vi "Railway-Crossing_vFinal_1.vi"() -> ()   [LabVIEW 2021]
uses:
  <vilib>/Utility/error.llb/DialogType.ctl
  <vilib>/DAQmx/write.llb/DAQmx Write (Counter Frequency 1Chan 1Samp).vi
  <vilib>/DAQmx/create/channels.llb/DAQmx Create Channel (CO-Pulse Generation-Frequency).vi
  <vilib>/DAQmx/configure/timing.llb/DAQmx Timing (Implicit).vi
  <vilib>/DAQmx/miscellaneous.llb/DAQmx Fill In Error Info.vi
panel:
  in  "stop 2":bool caption="stop"
  out "Car Counter 2":dbl
  out "Peak/Off-Peak":bool
  out "Car Counter":dbl
  out "Elapsed Time":dbl format="%#.0p"
  out "Time of Day":string
  out "Servo 2":bool
  out "Servo":bool
  in  "stop":bool
  out "Train":bool
  out "Train 2":bool
  out "Trainf":bool
  out "GREEN 2":bool
  out "YELLOW 2":bool
  out "RED  2":bool
  out "GREEN 1":bool
  out "YELLOW 1":bool
  out "GREEN":bool
  out "YELLOW":bool
  out "RED1":bool
  out "RED":bool
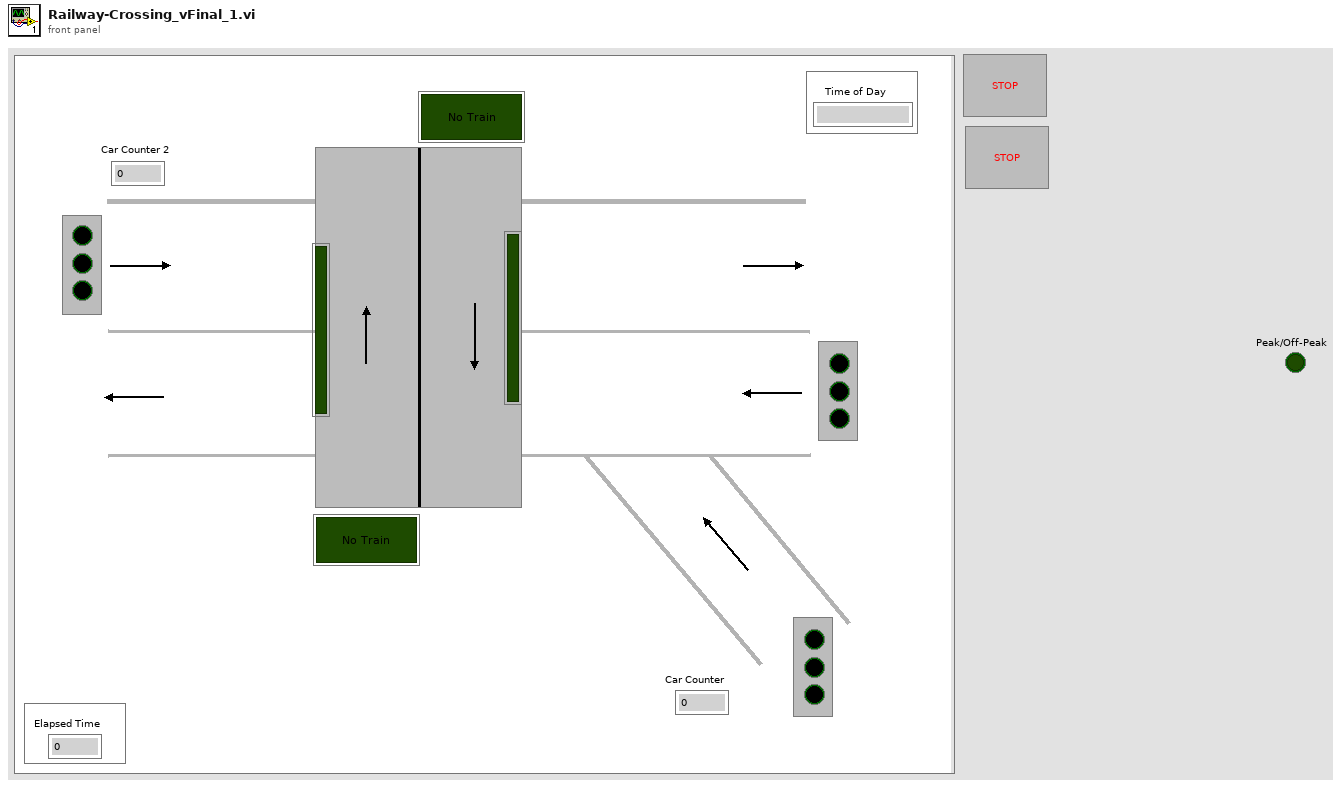
[diagram p1: front panel]
types:
  T1 = typedef "DialogType.ctl" = u16
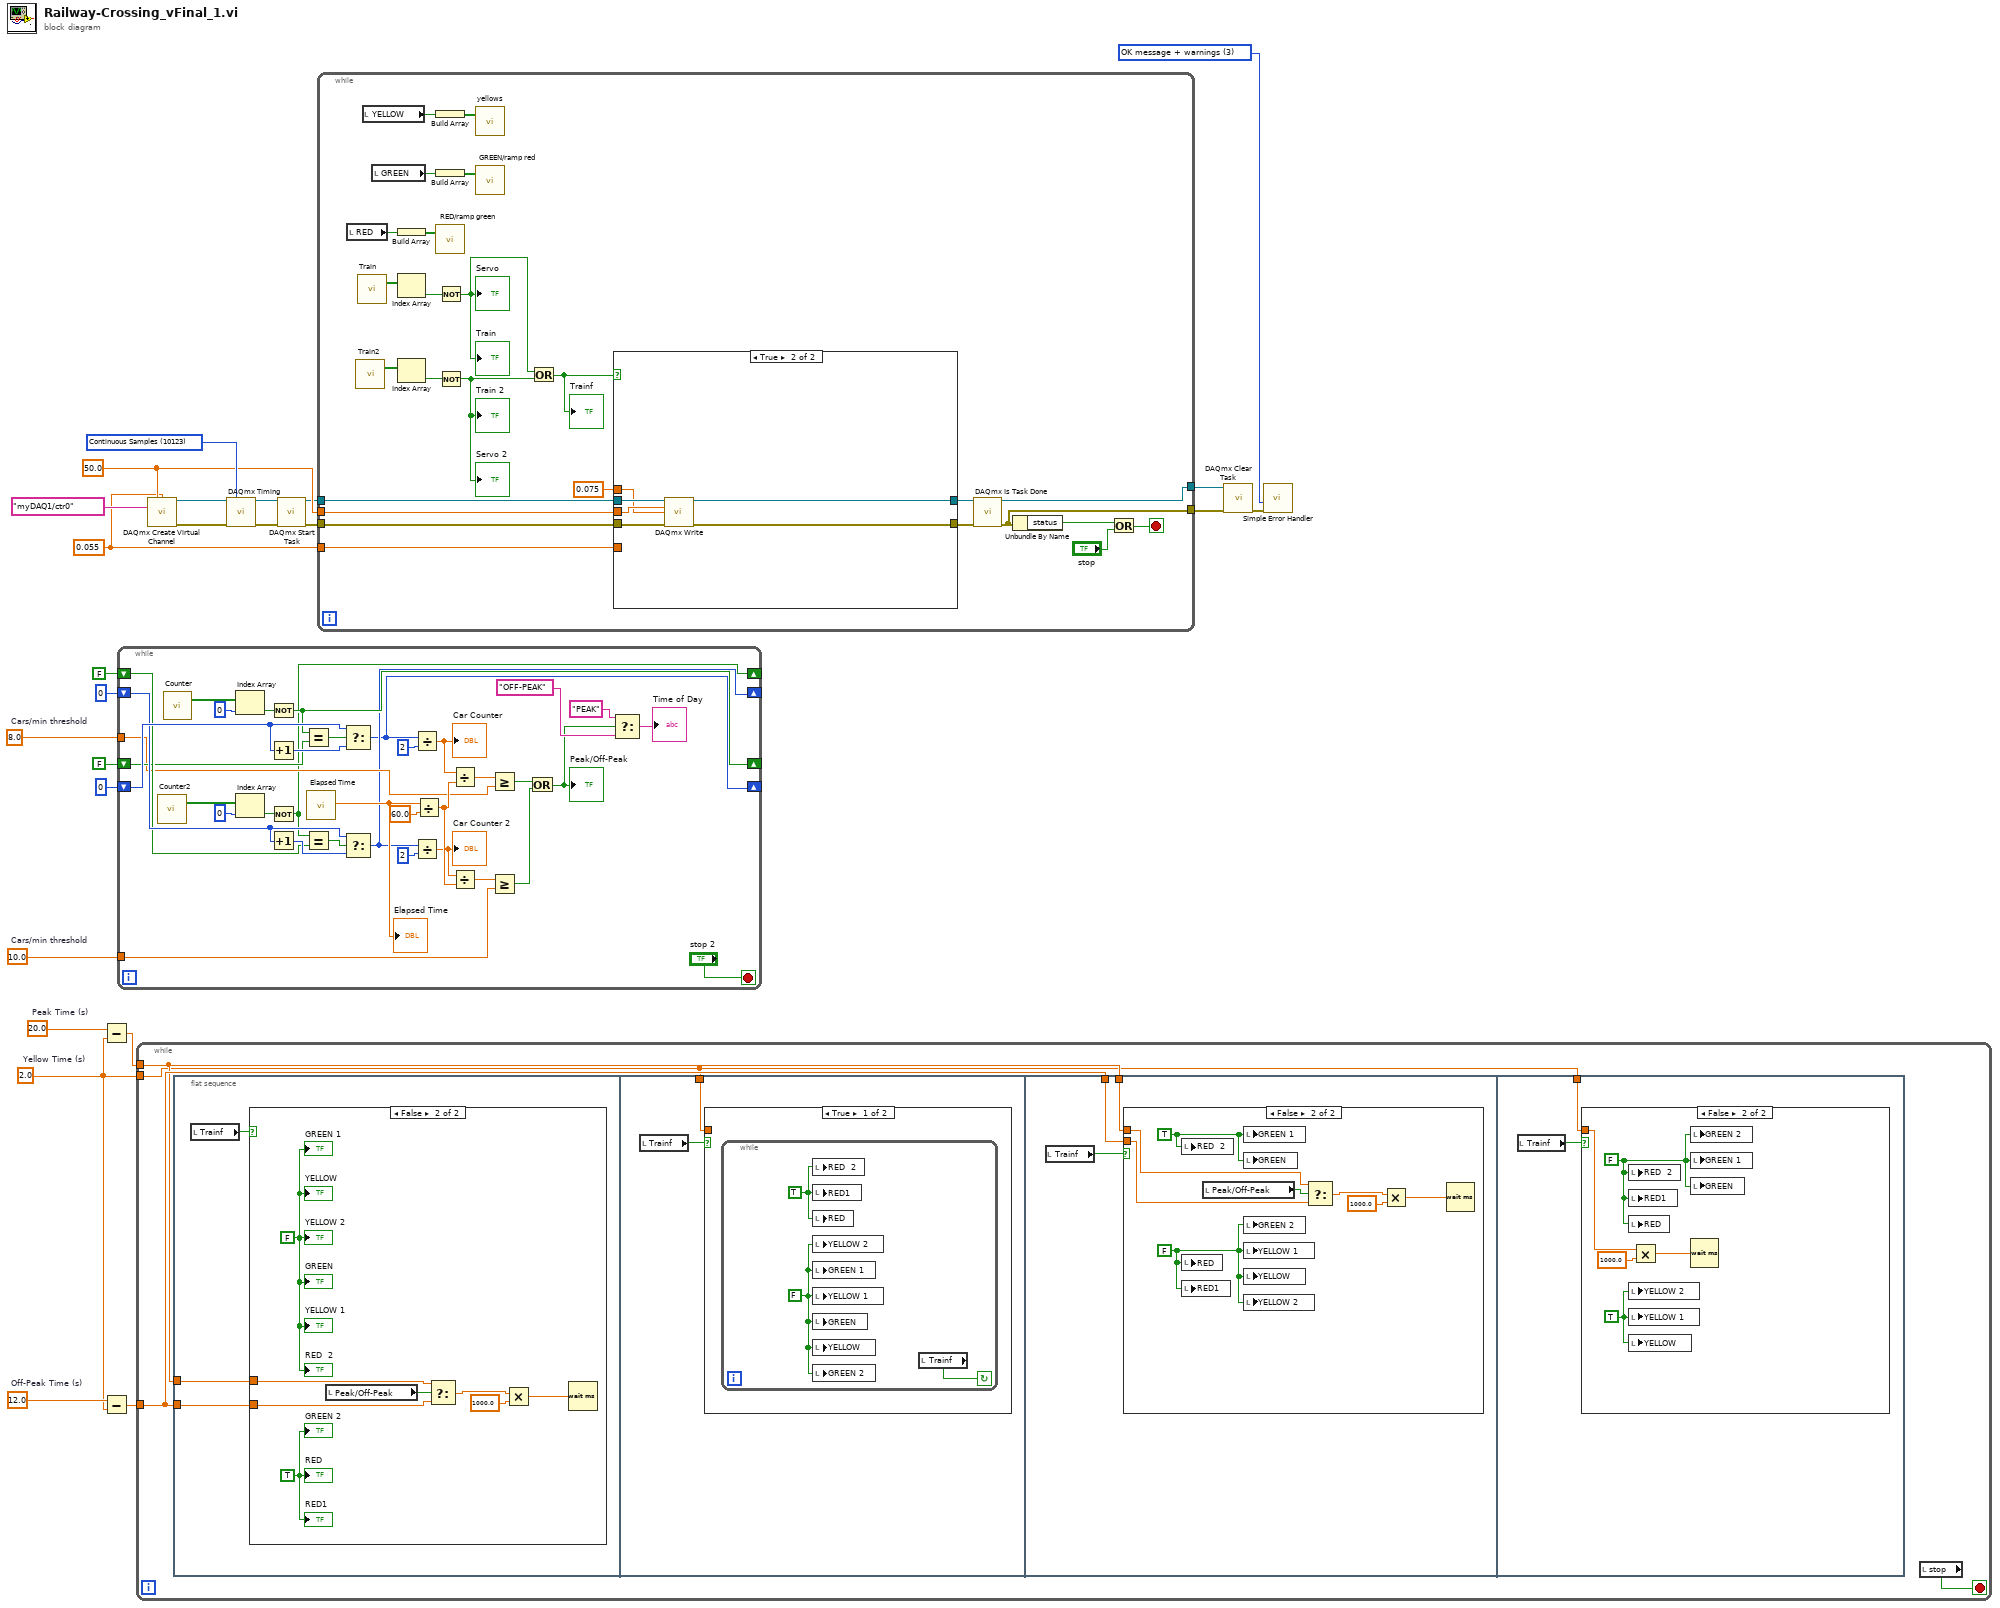
[diagram p0: block diagram]
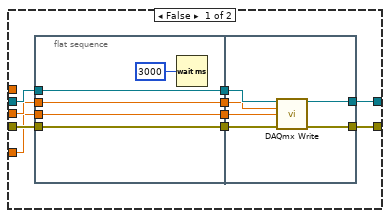
[diagram p2: hidden frame]
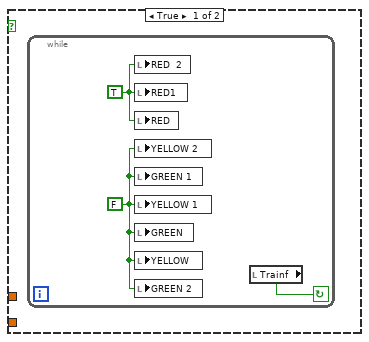
[diagram p3: hidden frame]
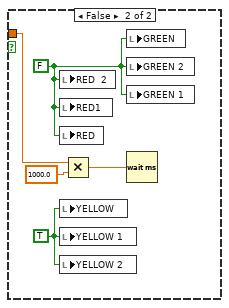
[diagram p4: hidden frame]
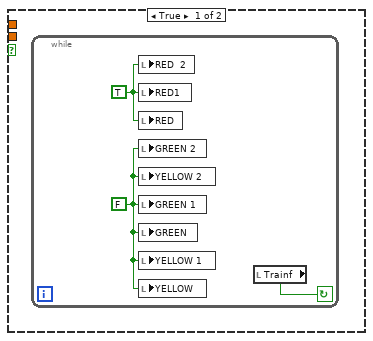
[diagram p5: hidden frame]
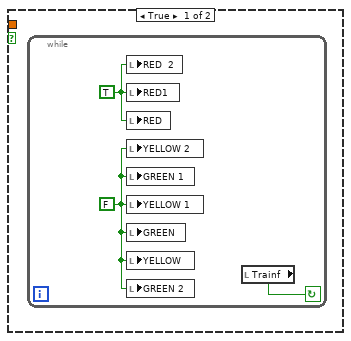
[diagram p6: hidden frame]
diagram:
  w2 = 10.0  # Cars/min threshold
  w1 = 8.0  # Cars/min threshold
  w10 = T1 3 items=["no dialog", "OK message", "continue or stop message", "OK message + warnings", "continue/stop + warnings"] ("type of dialog (OK msg:1)")
  w7 = 0.055 ("Duty Cycle")
  w14 = 50.0 ("Frequency")
  w16 = 10123 items=["Finite Samples"=10178, "Continuous Samples"=10123] ("sample mode")
  w23 = 20.0  # Peak Time (s)
  w22 = 2.0  # Yellow Time (s)
  w24 = 12.0  # Off-Peak Time (s)
  n1 = Subtract(x=w23, y=w22) -> (x-y=w21:dbl)
  n2 = Subtract(x=w24, y=w22) -> (x-y=w25:dbl)
  n3 = while {
    shift-right: [w32] -> _
    shift-left: FALSE -> [w37]
    shift-right: [w31] -> _
    shift-left: 0 -> [w38]
    shift-right: [w33] -> _
    shift-left: FALSE -> [w36]
    shift-right: [w27] -> _
    shift-left: 0 -> [w39]
    tunnel: w2 -> [w35]
    tunnel: w1 -> [w34]
    stop <- "stop 2" stop-if-true
    n4 = call "Counter2"() -> ("data"=w53:bool[])  [unwired: 17 in, 2 out]
    n5 = call "Counter"() -> ("data"=w56:bool[])  [unwired: 17 in, 2 out]
    n6 = Index Array(array=w56, index=0) -> (element=w55:bool)
    n7 = Index Array(array=w53, index=0) -> (element=w52:bool)
    n8 = Not(x=w55) -> (.not. x?=w33:bool)
    n9 = Increment(x=w39) -> (x+1=w54:i32)
    n10 = Not(x=w52) -> (.not. x?=w32:bool)
    n11 = Increment(x=w38) -> (x+1=w51:i32)
    n12 = Equal?(x=w33, y=w36) -> (x = y?=w44:bool)
    n13 = Equal?(x=w32, y=w37) -> (x = y?=w41:bool)
    n14 = call "Elapsed Time"() -> ("Elapsed Time (s)"=w61:dbl)  [unwired: 12 in, 7 out]
    "Elapsed Time" <- w61
    n15 = Select(t=w39, s=w44, f=w54) -> (s? t:f=w27:i32)
    n16 = Select(t=w38, s=w41, f=w51) -> (s? t:f=w31:i32)
    n17 = Divide(x=w27, y=2) -> (x/y=w26:dbl)
    "Car Counter" <- w26
    n18 = Divide(x=w31, y=2) -> (x/y=w29:dbl)
    "Car Counter 2" <- w29
    n19 = Divide(x=w61, y=60.0) -> (x/y=w50:dbl)
    n20 = Divide(x=w26, y=w50) -> (x/y=w48:dbl)
    n21 = Divide(x=w29, y=w50) -> (x/y=w49:dbl)
    n22 = Greater Or Equal?(x=w48, y=w34) -> (x >= y?=w47:bool)
    n23 = Greater Or Equal?(x=w49, y=w35) -> (x >= y?=w46:bool)
    n24 = Or(x=w47, y=w46) -> (x .or. y?=w45:bool)
    "Peak/Off-Peak" <- w45
    n25 = Select(t="PEAK", s=w45, f="OFF-PEAK") -> (s? t:f=→"Time of Day":string)
  }
  n26 = while {
    tunnel: w22 -> [w62]
    tunnel: w25 -> [w65]
    tunnel: w21 -> [w64]
    stop <- w63 stop-if-true
    n27 = flat-sequence {
      tunnel: w65 -> [w68]
      tunnel: w64 -> [w67]
      tunnel: w62 -> [w81]
      tunnel: w65 -> [w92]
      tunnel: w64 -> [w91]
      tunnel: w62 -> [w105]
      frame #0 {
        n28 = local read "Trainf"() -> (w66:bool)
        n29 = case shown="False" w66 {
          tunnel: w68 -> [_ w76]
          tunnel: w67 -> [_ w74]
          frame True {
            n30 = while {
              stop <- w69 continue-if-true
              w70 = FALSE ("GREEN 2")
              w71 = TRUE ("RED1")
              n31 = local write "RED  2"(w71) -> ()
              n32 = local write "RED1"(w71) -> ()
              n33 = local write "RED"(w71) -> ()
              n34 = local write "YELLOW 2"(w70) -> ()
              n35 = local write "GREEN 1"(w70) -> ()
              n36 = local write "YELLOW 1"(w70) -> ()
              n37 = local write "GREEN"(w70) -> ()
              n38 = local write "YELLOW"(w70) -> ()
              n39 = local write "GREEN 2"(w70) -> ()
              n40 = local read "Trainf"() -> (w69:bool)
            }
          }
          frame False {
            w72 = FALSE ("YELLOW")
            w73 = TRUE ("RED")
            n41 = local read "Peak/Off-Peak"() -> (w77:bool)
            n42 = Select(t=w74, s=w77, f=w76) -> (s? t:f=w75:dbl)
            n43 = Multiply(x=w75, y=1000.0) -> (x*y=w79:dbl)
            n44 = Wait (ms)(milliseconds to wait=w79) -> ()  [unwired: 1 out]
            "RED" <- w73
            "RED1" <- w73
            "YELLOW" <- w72
            "GREEN" <- w72
            "YELLOW 1" <- w72
            "GREEN 1" <- w72
            "RED  2" <- w72
            "YELLOW 2" <- w72
            "GREEN 2" <- w73
          }
        }
      }
      frame #1 {
        n45 = local read "Trainf"() -> (w80:bool)
        n46 = case shown="True" w80 {
          tunnel: w81 -> [_ w87]
          frame True {
            n47 = while {
              stop <- w83 continue-if-true
              w82 = FALSE ("GREEN")
              w84 = TRUE ("RED1  2")
              n48 = local write "RED  2"(w84) -> ()
              n49 = local write "RED1"(w84) -> ()
              n50 = local write "RED"(w84) -> ()
              n51 = local write "YELLOW 2"(w82) -> ()
              n52 = local write "GREEN 1"(w82) -> ()
              n53 = local write "YELLOW 1"(w82) -> ()
              n54 = local write "GREEN"(w82) -> ()
              n55 = local write "YELLOW"(w82) -> ()
              n56 = local write "GREEN 2"(w82) -> ()
              n57 = local read "Trainf"() -> (w83:bool)
            }
          }
          frame False {
            w86 = FALSE ("GREEN 2")
            w85 = TRUE ("RED")
            n58 = local write "RED  2"(w86) -> ()
            n59 = local write "RED1"(w86) -> ()
            n60 = local write "RED"(w86) -> ()
            n61 = local write "YELLOW"(w85) -> ()
            n62 = local write "YELLOW 1"(w85) -> ()
            n63 = local write "YELLOW 2"(w85) -> ()
            n64 = Multiply(x=w87, y=1000.0) -> (x*y=w89:dbl)
            n65 = local write "GREEN"(w86) -> ()
            n66 = local write "GREEN 2"(w86) -> ()
            n67 = local write "GREEN 1"(w86) -> ()
            n68 = Wait (ms)(milliseconds to wait=w89) -> ()  [unwired: 1 out]
          }
        }
      }
      frame #2 {
        n69 = local read "Trainf"() -> (w90:bool)
        n70 = case shown="False" w90 {
          tunnel: w92 -> [_ w98]
          tunnel: w91 -> [_ w96]
          frame True {
            n71 = while {
              stop <- w95 continue-if-true
              w93 = FALSE ("YELLOW")
              w94 = TRUE ("RED1  2")
              n72 = local write "RED  2"(w94) -> ()
              n73 = local write "RED1"(w94) -> ()
              n74 = local write "RED"(w94) -> ()
              n75 = local write "GREEN 2"(w93) -> ()
              n76 = local write "YELLOW 2"(w93) -> ()
              n77 = local write "GREEN 1"(w93) -> ()
              n78 = local write "GREEN"(w93) -> ()
              n79 = local write "YELLOW 1"(w93) -> ()
              n80 = local write "YELLOW"(w93) -> ()
              n81 = local read "Trainf"() -> (w95:bool)
            }
          }
          frame False {
            w100 = FALSE ("YELLOW")
            w101 = TRUE ("GREEN 2")
            n82 = local write "RED  2"(w101) -> ()
            n83 = local write "RED"(w100) -> ()
            n84 = local write "RED1"(w100) -> ()
            n85 = local read "Peak/Off-Peak"() -> (w99:bool)
            n86 = local write "GREEN 1"(w101) -> ()
            n87 = local write "GREEN"(w101) -> ()
            n88 = local write "GREEN 2"(w100) -> ()
            n89 = local write "YELLOW 1"(w100) -> ()
            n90 = local write "YELLOW"(w100) -> ()
            n91 = local write "YELLOW 2"(w100) -> ()
            n92 = Select(t=w96, s=w99, f=w98) -> (s? t:f=w97:dbl)
            n93 = Multiply(x=w97, y=1000.0) -> (x*y=w103:dbl)
            n94 = Wait (ms)(milliseconds to wait=w103) -> ()  [unwired: 1 out]
          }
        }
      }
      frame #3 {
        n95 = local read "Trainf"() -> (w104:bool)
        n96 = case shown="False" w104 {
          tunnel: w105 -> [_ w109]
          frame True {
            n97 = while {
              stop <- w108 continue-if-true
              w106 = TRUE ("RED1")
              w107 = FALSE ("GREEN 2")
              n98 = local write "RED  2"(w106) -> ()
              n99 = local write "RED1"(w106) -> ()
              n100 = local write "RED"(w106) -> ()
              n101 = local write "YELLOW 2"(w107) -> ()
              n102 = local write "GREEN 1"(w107) -> ()
              n103 = local write "YELLOW 1"(w107) -> ()
              n104 = local write "GREEN"(w107) -> ()
              n105 = local write "YELLOW"(w107) -> ()
              n106 = local write "GREEN 2"(w107) -> ()
              n107 = local read "Trainf"() -> (w108:bool)
            }
          }
          frame False {
            w110 = FALSE ("RED1")
            w111 = TRUE ("YELLOW 2")
            n108 = local write "RED  2"(w110) -> ()
            n109 = local write "RED1"(w110) -> ()
            n110 = local write "RED"(w110) -> ()
            n111 = local write "YELLOW 2"(w111) -> ()
            n112 = local write "YELLOW 1"(w111) -> ()
            n113 = local write "YELLOW"(w111) -> ()
            n114 = Multiply(x=w109, y=1000.0) -> (x*y=w113:dbl)
            n115 = local write "GREEN 2"(w110) -> ()
            n116 = local write "GREEN 1"(w110) -> ()
            n117 = local write "GREEN"(w110) -> ()
            n118 = Wait (ms)(milliseconds to wait=w113) -> ()  [unwired: 1 out]
          }
        }
      }
    }
    n119 = local read "stop"() -> (w63:bool)
  }
  n120 = call-poly <vilib>:"DAQmx Create Virtual Channel.vi"("frequency"=w14, "duty cycle"=w7, "counter"=tag "myDAQ1/ctr0" ("Counter(s)")) -> ("task out"=w19:refnum<k21>, "error out"=w20:errorcluster)  [unwired: 11 in]
  n121 = call-poly <vilib>:"DAQmx Timing.vi"("task/channels in"=w19, "sample mode"=w16, "error in"=w20) -> ("task out"=w17:refnum<k21>, "error out"=w18:errorcluster)  [unwired: 11 in]
  n122 = call <vilib>:"DAQmx Start Task.vi"("task/channels in"=w17, "error in"=w18) -> ("task out"=w13:refnum<k21>, "error out"=w12:errorcluster)  [unwired: 12 in]
  n123 = while {
    tunnel: w13 -> [w127]
    tunnel: w12 -> [w126]
    tunnel: w14 -> [w125]
    tunnel: [w124] -> w8
    tunnel: [w123] -> w9
    tunnel: w7 -> [w122]
    stop <- w128 stop-if-true
    n124 = local read "RED"() -> (w138:bool)
    n125 = call "Train2"() -> ("data"=w120:bool[])  [unwired: 17 in, 2 out]
    n126 = call "Train"() -> ("data"=w135:bool[])  [unwired: 17 in, 2 out]
    n127 = local read "YELLOW"() -> (w114:bool)
    n128 = local read "GREEN"() -> (w136:bool)
    n129 = Build Array(w138) -> (w116:bool[])
    n130 = Index Array(array=w135) -> (element=w134:bool)  [unwired: 1 in]
    n131 = Index Array(array=w120) -> (element=w121:bool)  [unwired: 1 in]
    n132 = Build Array(w114) -> (w115:bool[])
    n133 = Build Array(w136) -> (w137:bool[])
    n134 = call "RED/ramp green"("data"=w116) -> ()  [unwired: 17 in, 2 out]
    n135 = Not(x=w134) -> (.not. x?=w119:bool)
    "Train" <- w119
    "Servo" <- w119
    n136 = Not(x=w121) -> (.not. x?=w118:bool)
    "Train 2" <- w118
    "Servo 2" <- w118
    n137 = call "yellows"("data"=w115) -> ()  [unwired: 17 in, 2 out]
    n138 = call "GREEN/ramp red"("data"=w137) -> ()  [unwired: 17 in, 2 out]
    n139 = Or(x=w119, y=w118) -> (x .or. y?=w117:bool)
    "Trainf" <- w117
    n140 = case shown="True" w117 {
      tunnel: [w146 w161] -> w131
      tunnel: [w145 w160] -> w130
      tunnel: w127 -> [w148 w165]
      tunnel: w126 -> [w147 w162]
      tunnel: w125 -> [w144 w164]
      tunnel: 0.075 ("Duty Cycle") -> [_ w163]
      tunnel: w122 -> [w143 _]
      frame False {
        n141 = flat-sequence {
          tunnel: w143 -> [w150]
          tunnel: w144 -> [w151]
          tunnel: w147 -> [w152]
          tunnel: w148 -> [w153]
          tunnel: [w153] -> w142
          tunnel: [w152] -> w141
          tunnel: [w151] -> w140
          tunnel: [w150] -> w139
          tunnel: [w157] -> w146
          tunnel: [w156] -> w145
          tunnel: w142 -> [w159]
          tunnel: w141 -> [w158]
          tunnel: w140 -> [w155]
          tunnel: w139 -> [w154]
          frame #0 {
            n142 = Wait (ms)(milliseconds to wait=3000) -> ()  [unwired: 1 out]
          }
          frame #1 {
            n143 = call-poly <vilib>:"DAQmx Write.vi"("task/channels in"=w159, "frequency"=w155, "duty cycle"=w154, "error in"=w158) -> ("task out"=w157:refnum<k21>, "error out"=w156:errorcluster)  [unwired: 9 in, 1 out]
          }
        }
      }
      frame True {
        n144 = call-poly <vilib>:"DAQmx Write.vi"("task/channels in"=w165, "frequency"=w164, "duty cycle"=w163, "error in"=w162) -> ("task out"=w161:refnum<k21>, "error out"=w160:errorcluster)  [unwired: 9 in, 1 out]
      }
    }
    n145 = call <vilib>:"DAQmx Is Task Done.vi"("task/channels in"=w131, "error in"=w130) -> ("task out"=w123:refnum<k21>, "error out"=w124:errorcluster)  [unwired: 11 in, 1 out]
    n146 = Unbundle By Name(w124) -> ("status"=w133:bool)
    n147 = Or(x=w133, y="stop") -> (x .or. y?=w128:bool)
  }
  n148 = call <vilib>:"DAQmx Clear Task.vi"("task in"=w9, "error in"=w8) -> ("error out"=w11:errorcluster)  [unwired: 13 in]
  n149 = call <vilib>:"Simple Error Handler.vi"("type of dialog (OK msg:1)"=w10, "error in (no error)"=w11) -> ()  [unwired: 3 in, 5 out]
